vi "laserStatus.vi"(8 "error in (no error)":errorcluster, 11 "VISA resource name":refnum<visa-resource-name>) -> (0 "error out":errorcluster, 3 "?":T1)   [LabVIEW 2013]
panel:
  out "LaserEnergy uJ":dbl
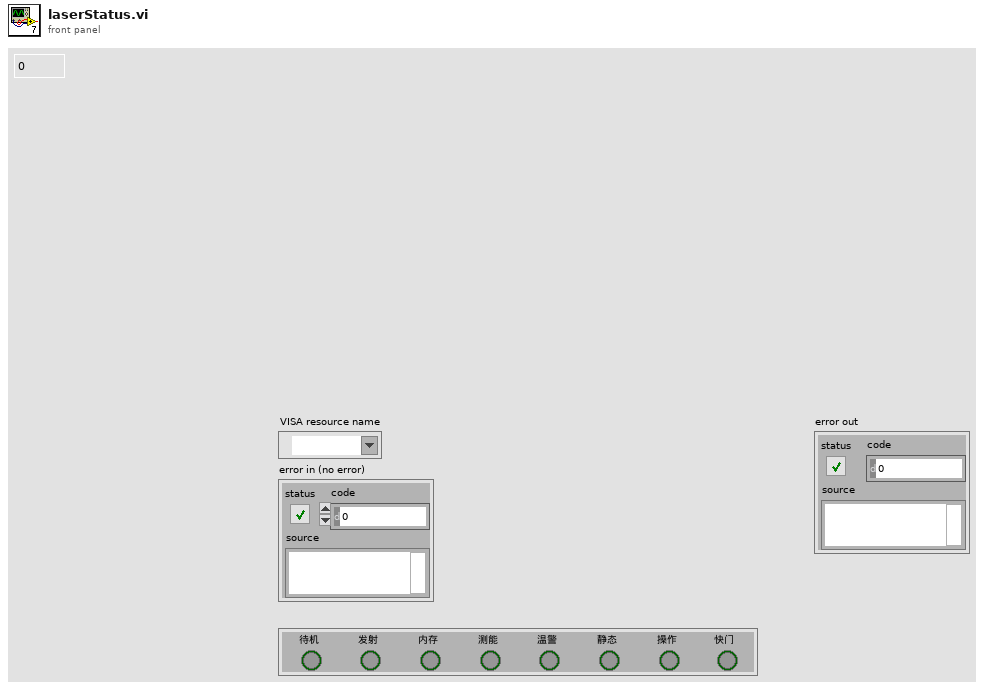
[diagram p1: front panel]
types:
  T1 = cluster{"待机":bool, "发射":bool, "内存":bool, "测能":bool, "温警":bool, "静态":bool, "操作":bool, "快门":bool}
  T2 = cluster{bool, bool, bool, bool, bool, bool, bool, bool}
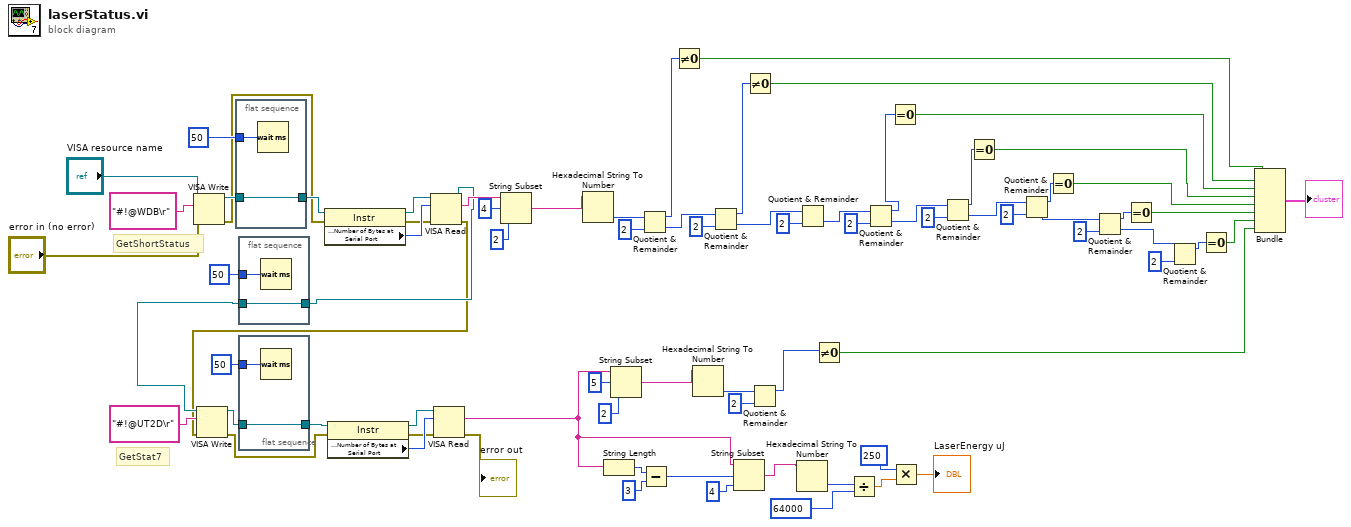
[diagram p0: block diagram]
diagram:
  # "GetStat7"
  # "GetShortStatus"
  n1 = VISA Write(VISA resource name="VISA resource name", write buffer="#!@WDB\r", error in (no error)="error in (no error)") -> (VISA resource name out=w71:refnum<visa-resource-name>, error out=w5:errorcluster)  [unwired: 1 out]
  n2 = flat-sequence {
    tunnel: w71 -> [w77]
    tunnel: [w77] -> w72
    tunnel: u32 50 ("delay before read (ms)") -> [w78]
    frame #0 {
      n3 = Wait (ms)(milliseconds to wait=w78) -> ()  [unwired: 1 out]
    }
  }
  n4 = flat-sequence {
    tunnel: [w79] -> w8
    tunnel: w9 -> [w79]
    tunnel: u32 50 ("delay before read (ms)") -> [w80]
    frame #0 {
      n5 = Wait (ms)(milliseconds to wait=w80) -> ()  [unwired: 1 out]
    }
  }
  n6 = flat-sequence {
    tunnel: w30 -> [w81]
    tunnel: [w81] -> w31
    tunnel: u32 50 ("delay before read (ms)") -> [w82]
    frame #0 {
      n7 = Wait (ms)(milliseconds to wait=w82) -> ()  [unwired: 1 out]
    }
  }
  n8 = property class="Instr"(reference=w72, error in=w5) -> (reference out=w73:refnum<visa-resource-name>, error out=w74:errorcluster, "Serial Settings:Number of Bytes at Serial Port"=w75:u32)
  n9 = VISA Read(VISA resource name=w73, byte count=w75, error in (no error)=w74) -> (VISA resource name out=w9:refnum<visa-resource-name>, read buffer=w69:string, error out=w4:errorcluster)  [unwired: 1 out]
  n10 = VISA Write(VISA resource name=w8, write buffer="#!@UT2D\r", error in (no error)=w4) -> (VISA resource name out=w30:refnum<visa-resource-name>, error out=w3:errorcluster)  [unwired: 1 out]
  n11 = property class="Instr"(reference=w31, error in=w3) -> (reference out=w32:refnum<visa-resource-name>, error out=w33:errorcluster, "Serial Settings:Number of Bytes at Serial Port"=w34:u32)
  n12 = VISA Read(VISA resource name=w32, byte count=w34, error in (no error)=w33) -> (read buffer=w17:string, error out=→"error out":errorcluster)  [unwired: 2 out]
  n13 = String Subset(string=w69, offset (0)=4, length (rest)=2 ("length (rest)")) -> (substring=w66:string)
  n14 = Hexadecimal String To Number(string=w66) -> (number=w65:u32)  [unwired: 2 in, 1 out]
  n15 = String Length(string=w17) -> (length=w20:i32)
  n16 = String Subset(string=w17, offset (0)=5, length (rest)=2 ("length (rest)")) -> (substring=w26:string)
  n17 = Quotient & Remainder(x=w65, y=2) -> (x-y*floor(x/y)=w63:u32, floor(x/y)=w60:u32)
  n18 = Subtract(x=w20, y=3) -> (x-y=w18:i32)
  n19 = Not Equal To 0?(x=w63) -> (x != 0?=w42:bool)
  n20 = Hexadecimal String To Number(string=w26) -> (number=w25:u32)  [unwired: 2 in, 1 out]
  n21 = Quotient & Remainder(x=w60, y=2) -> (x-y*floor(x/y)=w61:u32, floor(x/y)=w58:u32)
  n22 = String Subset(string=w17, offset (0)=w18, length (rest)=4) -> (substring=w15:string)
  n23 = Not Equal To 0?(x=w61) -> (x != 0?=w41:bool)
  n24 = Quotient & Remainder(x=w25, y=2) -> (x-y*floor(x/y)=w22:u32)  [unwired: 1 out]
  n25 = Hexadecimal String To Number(string=w15) -> (number=w14:u32)  [unwired: 2 in, 1 out]
  n26 = Quotient & Remainder(x=w58, y=2) -> (floor(x/y)=w56:u32)  [unwired: 1 out]
  n27 = Not Equal To 0?(x=w22) -> (x != 0?=w21:bool)
  n28 = Divide(x=w14, y=u32 64000) -> (x/y=w12:dbl)
  n29 = Quotient & Remainder(x=w56, y=2) -> (x-y*floor(x/y)=w55:u32, floor(x/y)=w53:u32)
  n30 = Equal To 0?(x=w55) -> (x = 0?=w40:bool)
  n31 = Multiply(x=250, y=w12) -> (x*y=→"LaserEnergy uJ":dbl)
  n32 = Quotient & Remainder(x=w53, y=2) -> (x-y*floor(x/y)=w52:u32, floor(x/y)=w49:u32)
  n33 = Equal To 0?(x=w52) -> (x = 0?=w39:bool)
  n34 = Quotient & Remainder(x=w49, y=2) -> (x-y*floor(x/y)=w50:u32, floor(x/y)=w46:u32)
  n35 = Equal To 0?(x=w50) -> (x = 0?=w38:bool)
  n36 = Quotient & Remainder(x=w46, y=2) -> (x-y*floor(x/y)=w47:u32, floor(x/y)=w43:u32)
  n37 = Equal To 0?(x=w47) -> (x = 0?=w37:bool)
  n38 = Quotient & Remainder(x=w43, y=2) -> (x-y*floor(x/y)=w44:u32)  [unwired: 1 out]
  n39 = Equal To 0?(x=w44) -> (x = 0?=w36:bool)
  n40 = Bundle(w42, w41, w40, w39, w38, w37, w36, w21) -> (→"?":T2)  [unwired: 1 in]
